vi "SwerveNewAngle.vi"(6 "String":string="RR Steer", 7 "Request Angle":dbl, 10 "Current Position":dbl) -> (2 "Set Position":dbl)   [LabVIEW 2016]
uses:
  Robot Global Data.vi
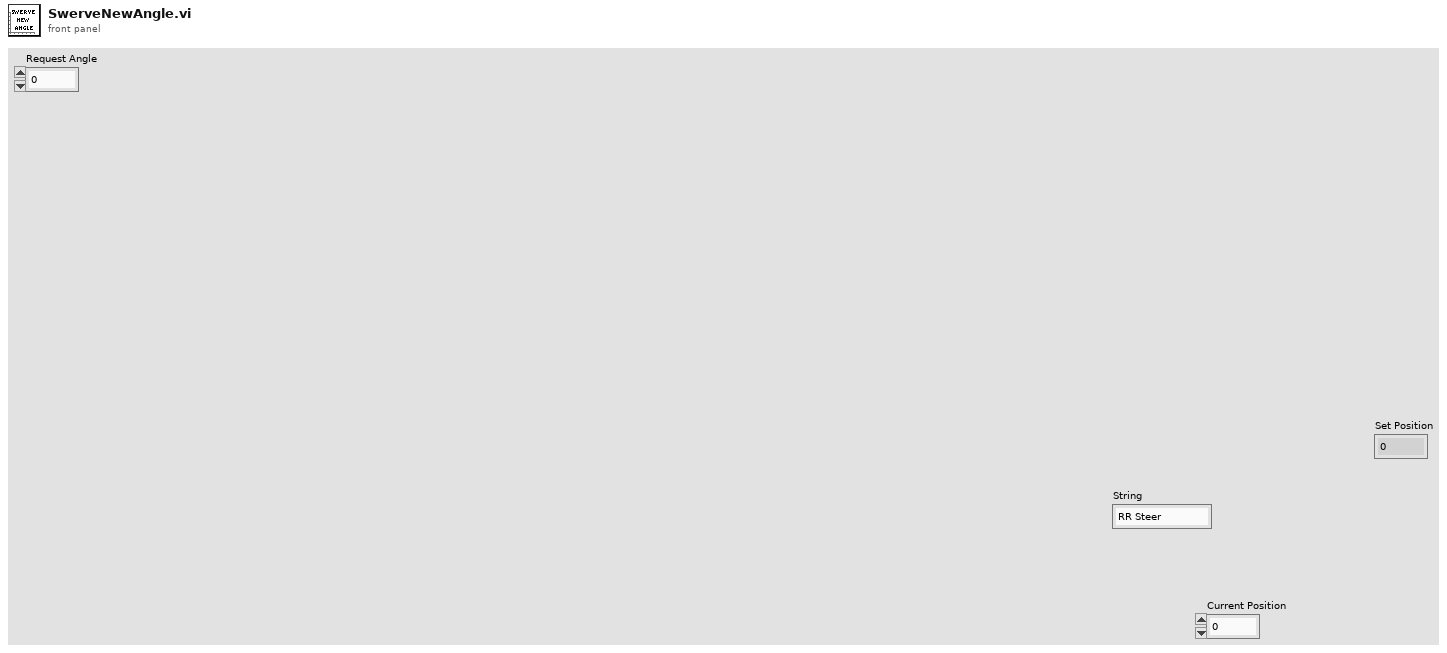
[diagram p1: front panel]
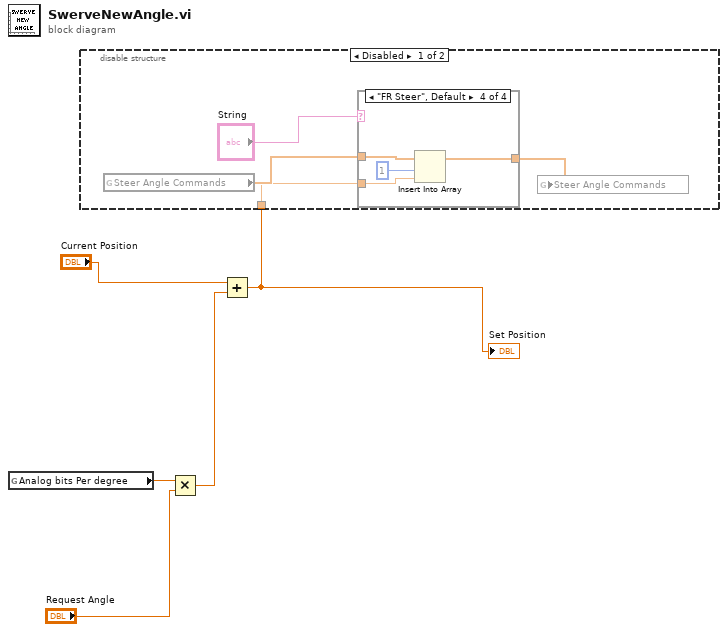
[diagram p0: block diagram]
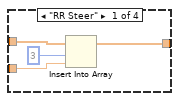
[diagram p2: hidden frame]
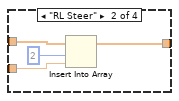
[diagram p3: hidden frame]
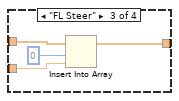
[diagram p4: hidden frame]
diagram:
  n1 = global read "Robot Global Data.vi" "Analog bits Per degree"() -> (w4:dbl)
  n2 = Multiply(x=w4, y="Request Angle") -> (x*y=w3:dbl)
  n3 = Add(x="Current Position", y=w3) -> (x+y=w5:dbl)
  "Set Position" <- w5
  n4 = disable-structure shown="Disabled" {
    disable-tunnel: w5 -> [w6 _]
    frame Disabled {
      n5 = global read "Robot Global Data.vi" "Steer Angle Commands"() -> (w8:dbl[])
      n6 = case shown="\"FR Steer\", Default" "String" {
        tunnel: w6 -> [w12 w15 w20 w24]
        tunnel: w8 -> [w13 w17 w21 w25]
        tunnel: [w11 w16 w19 w23] -> w7
        frame "RR Steer" {
          n7 = Insert Into Array "Insert Into Array"(array=w13, index=3, new element=w12) -> (w11:dbl[])
        }
        frame "RL Steer" {
          n8 = Insert Into Array(array=w17, index=2, new element=w15) -> (w16:dbl[])
        }
        frame "FL Steer" {
          n9 = Insert Into Array(array=w21, index=0, new element=w20) -> (w19:dbl[])
        }
        frame "FR Steer", Default {
          n10 = Insert Into Array(array=w25, index=1, new element=w24) -> (w23:dbl[])
        }
      }
      n11 = global write "Robot Global Data.vi" "Steer Angle Commands"(w7) -> ()
    }
    frame Enabled {
    }
  }
